vi "ttm_start.vi"() -> ()   [LabVIEW 2011]
panel:
  in  "ttm_twocreep_ramprate":dbl=0.001
  in  "ttm_twocreep_relaxationtime":dbl=30.0
  in  "ttm_twocreep_loadtime":dbl=30.0
  in  "ttm_twocreep_load":dbl=0.01
  in  "ttm_movetosetpoint_setpointtime":dbl=5.0
  in  "ttm_movetosetpoint_rampsetpoint":dbl
  in  "ttm_tensile_ramprate":dbl=0.01 step=0.001
  in  "ttm_tensile_rampamplitude":dbl=5000.0
  in  "ttm_tensile_channel":i32=1
  in  "ttm_aecontrol_channel":i32=1
  in  "ttm_aecontrol_rampratesilent":dbl=0.01 step=0.001
  in  "ttm_aecontrol_holdtime":dbl=5000.0
  in  "ttm_aecontrol_timewindow":dbl=1000.0
  in  "ttm_tensilecyclic_channel":dbl=1.0
  in  "ttm_tensilecyclic_separateloggings":bool=TRUE
  in  "ttm_tensilecyclic_ramptargetpressure":dbl=-700.0
  in  "ttm_tensilecyclic_zdim3":dbl=11.1
  in  "ttm_tensilecyclic_ydim3":dbl=11.1
  in  "ttm_tensilecyclic_xdim3":dbl=11.1
  in  "ttm_tensilecyclic_zdim2":dbl=11.1
  in  "ttm_tensilecyclic_ydim2":dbl=11.1
  in  "ttm_tensilecyclic_xdim2":dbl=11.1
  in  "ttm_tensilecyclic_zdim1":dbl=11.1
  in  "ttm_tensilecyclic_ydim1":dbl=11.1
  in  "ttm_tensilecyclic_xdim1":dbl=11.1
  in  "ttm_global_comment":string
  in  "ttm_tensilecyclic_timecycles":i32=10
  in  "ttm_tensilecyclic_timepreramp":i32=5
  in  "ttm_tensilecyclic_rampsetpoint":dbl=-0.04
  in  "ttm_tensilecyclic_numberofrounds":i32=2
  in  "ttm_tensilecyclic_cyclicfrequency":dbl=0.5
  in  "ttm_tensilecyclic_cyclicamplitude":dbl=0.05
  in  "ttm_global_expid":string="test"
  in  "ttm_global_parentfolder":string="C:\\Documents and Settings\\sauna\\Desktop\\MatleenaLabVIEW\\Testing\\"
  in  "ttm_aecontrol_targetvalue":dbl=1.0
  in  "aechangeofforcewithinbufferloop":dbl
  in  "ttm_aecontrol_aedatasum":dbl
  in  "ttm_aecontrol_initialforce":dbl
  in  "ttm_global_window":dbl
  in  "ttm_creep_channel":dbl=1.0
  in  "ttm_tensilecyclic_cyclicsetpoint":dbl=-0.1
  in  "ttm_aecontrol_ramprateae":dbl
  in  "ttm_global_protocol":string="tensilecyclic"
  in  "ttm_creep_load":dbl
  in  "ttm_tensilecyclic_ramprate":dbl=-0.01
  # "* = \"Put this negative if you are doing a compression experiment.\""
  # "*\n*\n*\n*\n*\n*\n*\n*\n*\n*\n*\n*\n*\n*\n*\n*\n*\n*\n*\n*"
  # "*"
  # "*"
  # "*"
  # "*"
  # "MEASUREMENTS AS MILLIMETERS"
  # "NOTE! \nDO NOT use double dots! (:)"
  # "***************************************"
  # "*\n*\n*\n*\n*\n*\n*\n*\n*\n*\n*\n*\n*\n*\n*"
  # "<-- \nPut negative values in these two  if you want to make compression (upper plate moving down).\n<---"
  # "<-- Separate ramp parts and cyclic parts into separate files"
  # "<-- Put all the data into the same file"
  # "***************************************"
  # "***************************************"
  # "*******************************"
  # "*\n*\n*\n*\n*\n*\n*\n*\n*\n*\n*\n*\n*\n*\n*"
  # "AE CONTROL"
  # "***************************************"
  # "mm/s"
  # "mm/s"
  # "ms"
  # "ms"
  # "AE control DEPRECATED?"
  # "How many events are needed within timewindow before changing to ramprateae"
  # "This actually is calculated in AE_data_read, initial value should be 0"
  # "1=position, 2=load, 3=digital position"
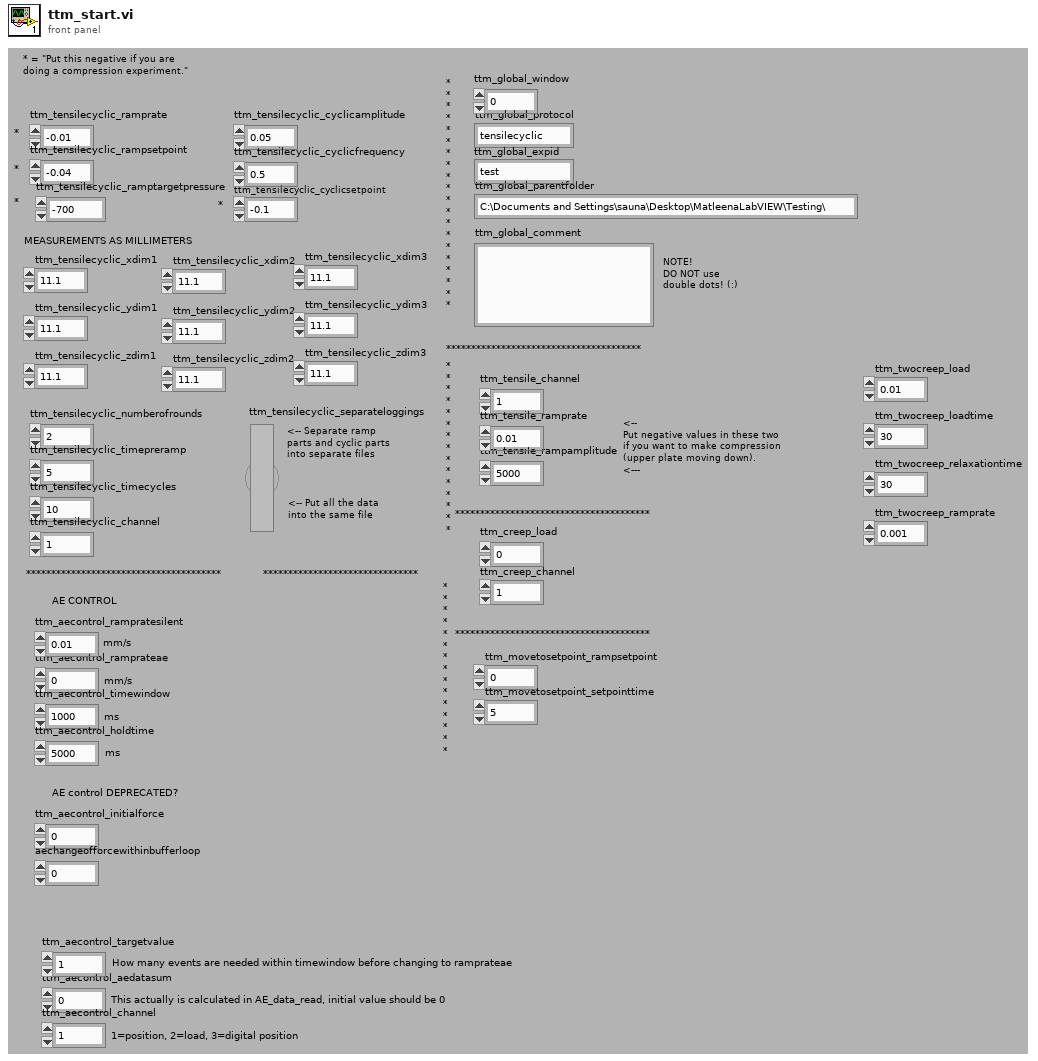
[diagram p1: front panel]
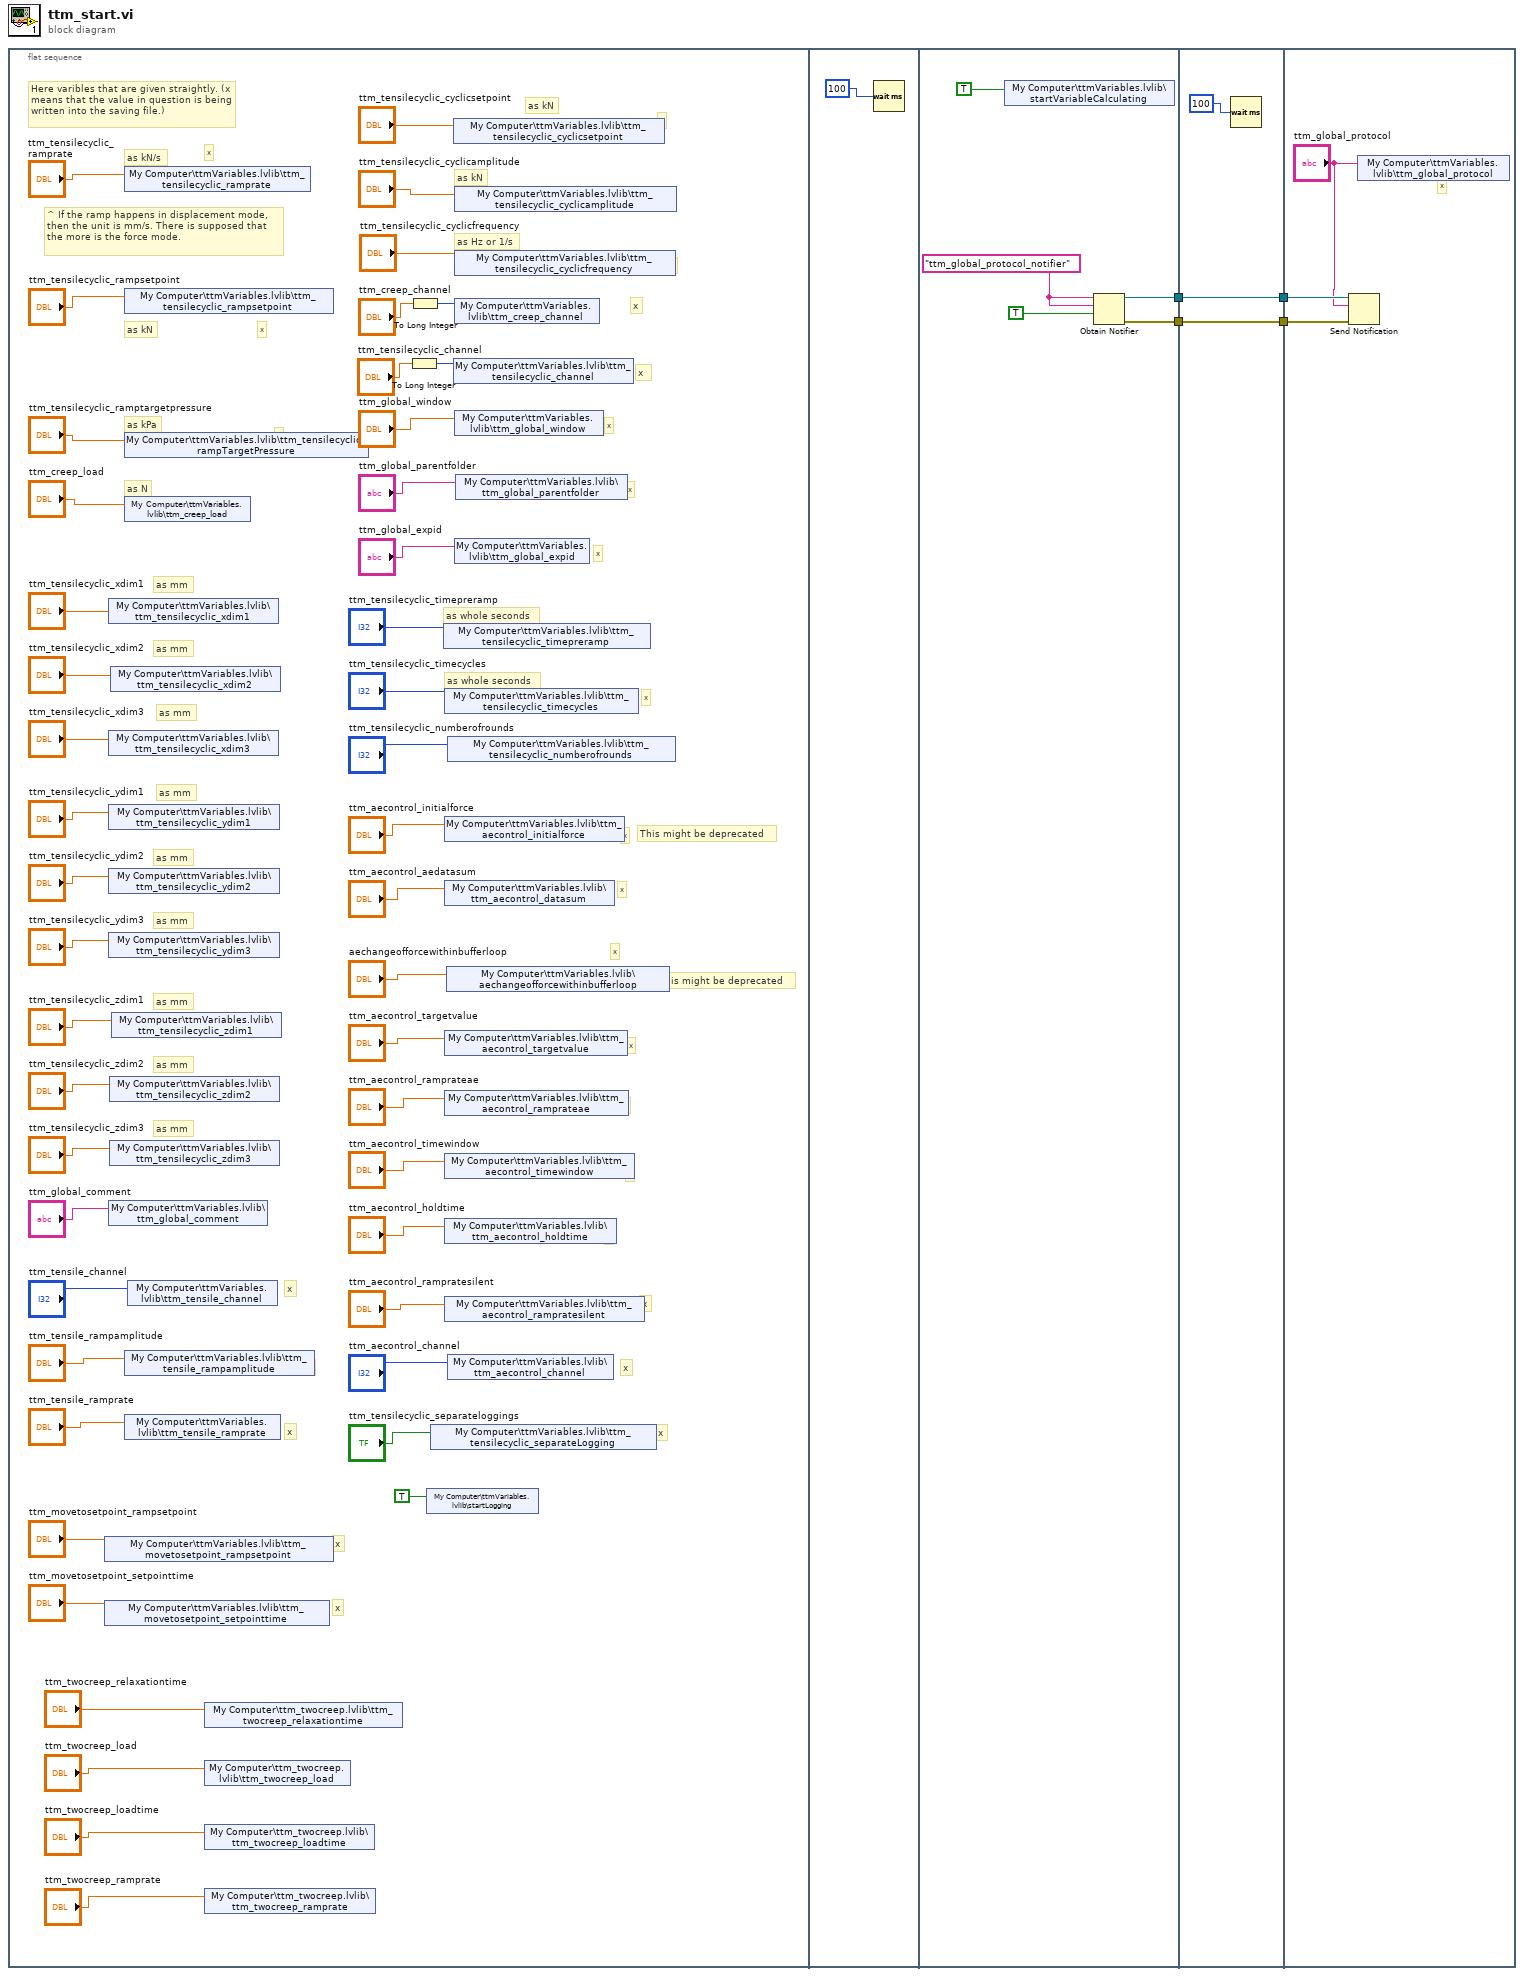
[diagram p0: block diagram]
diagram:
  n1 = flat-sequence {
    tunnel: [w54] -> w3
    tunnel: [w53] -> w1
    tunnel: [w59] -> w4
    tunnel: w3 -> [w59]
    tunnel: [w58] -> w2
    tunnel: w1 -> [w58]
    tunnel: w4 -> [w63]
    tunnel: w2 -> [w61]
    frame #0 {
      # "x"
      # "x"
      # "x"
      # "x"
      # "x"
      # "x"
      # "x"
      # "This might be deprecated"
      # "x"
      # "x"
      # "x"
      # "This might be deprecated"
      # "x"
      # "^ If the ramp happens in displacement mode, then the unit is mm/s. There is supposed that the more is the force mode."
      # "as kN"
      # "as Hz or 1/s"
      # "as N"
      # "as kN"
      # "as kN/s"
      # "as mm"
      # "as mm"
      # "as mm"
      # "as mm"
      # "as mm"
      # "as mm"
      # "as mm"
      # "as mm"
      # "as mm"
      # "as kN"
      # "as whole seconds"
      # "as whole seconds"
      # "Here varibles that are given straightly. (x means that the value in question is being written into the saving file.)"
      # "x"
      # "as kPa"
      # "x"
      # "x"
      # "x"
      # "x"
      # "x"
      # "x"
      # "x"
      # "x"
      # "x"
      # "x"
      # "x"
      # "x"
      # "x"
      # "x"
      # "x"
      # "x"
      # "x"
      # "x"
      # "x"
      n2 = shared-variable "My Computer\\ttmVariables.lvlib\\ttm_movetosetpoint_rampsetpoint"("ttm_movetosetpoint_rampsetpoint") -> ()  [unwired: 1 in, 1 out]
      n3 = shared-variable "My Computer\\ttmVariables.lvlib\\ttm_movetosetpoint_setpointtime"("ttm_movetosetpoint_setpointtime") -> ()  [unwired: 1 in, 1 out]
      n4 = shared-variable "My Computer\\ttmVariables.lvlib\\ttm_tensilecyclic_xdim1"("ttm_tensilecyclic_xdim1") -> ()  [unwired: 1 in, 1 out]
      n5 = shared-variable "My Computer\\ttmVariables.lvlib\\ttm_tensilecyclic_xdim3"("ttm_tensilecyclic_xdim3") -> ()  [unwired: 1 in, 1 out]
      n6 = shared-variable "My Computer\\ttmVariables.lvlib\\ttm_tensilecyclic_ydim1"("ttm_tensilecyclic_ydim1") -> ()  [unwired: 1 in, 1 out]
      n7 = shared-variable "My Computer\\ttmVariables.lvlib\\ttm_tensilecyclic_ydim2"("ttm_tensilecyclic_ydim2") -> ()  [unwired: 1 in, 1 out]
      n8 = shared-variable "My Computer\\ttmVariables.lvlib\\ttm_tensilecyclic_ydim3"("ttm_tensilecyclic_ydim3") -> ()  [unwired: 1 in, 1 out]
      n9 = shared-variable "My Computer\\ttmVariables.lvlib\\ttm_global_comment"("ttm_global_comment") -> ()  [unwired: 1 in, 1 out]
      n10 = shared-variable "My Computer\\ttmVariables.lvlib\\ttm_tensilecyclic_zdim2"("ttm_tensilecyclic_zdim2") -> ()  [unwired: 1 in, 1 out]
      n11 = shared-variable "My Computer\\ttmVariables.lvlib\\ttm_tensilecyclic_zdim3"("ttm_tensilecyclic_zdim3") -> ()  [unwired: 1 in, 1 out]
      n12 = shared-variable "My Computer\\ttmVariables.lvlib\\ttm_tensilecyclic_xdim2"("ttm_tensilecyclic_xdim2") -> ()  [unwired: 1 in, 1 out]
      n13 = shared-variable "My Computer\\ttmVariables.lvlib\\ttm_tensilecyclic_zdim1"("ttm_tensilecyclic_zdim1") -> ()  [unwired: 1 in, 1 out]
      n14 = shared-variable "My Computer\\ttmVariables.lvlib\\ttm_tensilecyclic_ramprate"("ttm_tensilecyclic_ramprate") -> ()  [unwired: 1 in, 1 out]
      n15 = shared-variable "My Computer\\ttmVariables.lvlib\\ttm_tensilecyclic_rampsetpoint"("ttm_tensilecyclic_rampsetpoint") -> ()  [unwired: 1 in, 1 out]
      n16 = shared-variable "My Computer\\ttmVariables.lvlib\\ttm_tensilecyclic_rampTargetPressure"("ttm_tensilecyclic_ramptargetpressure") -> ()  [unwired: 1 in, 1 out]
      n17 = shared-variable "My Computer\\ttmVariables.lvlib\\ttm_creep_load"("ttm_creep_load") -> ()  [unwired: 1 in, 1 out]
      n18 = shared-variable "My Computer\\ttmVariables.lvlib\\ttm_tensile_rampamplitude"("ttm_tensile_rampamplitude") -> ()  [unwired: 1 in, 1 out]
      n19 = shared-variable "My Computer\\ttmVariables.lvlib\\ttm_tensile_ramprate"("ttm_tensile_ramprate") -> ()  [unwired: 1 in, 1 out]
      n20 = shared-variable "My Computer\\ttmVariables.lvlib\\ttm_tensile_channel"("ttm_tensile_channel") -> ()  [unwired: 1 in, 1 out]
      n21 = shared-variable "My Computer\\ttm_twocreep.lvlib\\ttm_twocreep_relaxationtime"("ttm_twocreep_relaxationtime") -> ()  [unwired: 1 in, 1 out]
      n22 = shared-variable "My Computer\\ttm_twocreep.lvlib\\ttm_twocreep_load"("ttm_twocreep_load") -> ()  [unwired: 1 in, 1 out]
      n23 = shared-variable "My Computer\\ttm_twocreep.lvlib\\ttm_twocreep_loadtime"("ttm_twocreep_loadtime") -> ()  [unwired: 1 in, 1 out]
      n24 = shared-variable "My Computer\\ttm_twocreep.lvlib\\ttm_twocreep_ramprate"("ttm_twocreep_ramprate") -> ()  [unwired: 1 in, 1 out]
      n25 = To Long Integer(number="ttm_tensilecyclic_channel") -> (32bit integer=w19:i32)
      n26 = To Long Integer(number="ttm_creep_channel") -> (32bit integer=w32:i32)
      n27 = shared-variable "My Computer\\ttmVariables.lvlib\\startLogging"(TRUE ("startLogging")) -> ()  [unwired: 1 in, 1 out]
      n28 = shared-variable "My Computer\\ttmVariables.lvlib\\ttm_tensilecyclic_separateLogging"("ttm_tensilecyclic_separateloggings") -> ()  [unwired: 1 in, 1 out]
      n29 = shared-variable "My Computer\\ttmVariables.lvlib\\ttm_tensilecyclic_timepreramp"("ttm_tensilecyclic_timepreramp") -> ()  [unwired: 1 in, 1 out]
      n30 = shared-variable "My Computer\\ttmVariables.lvlib\\ttm_tensilecyclic_timecycles"("ttm_tensilecyclic_timecycles") -> ()  [unwired: 1 in, 1 out]
      n31 = shared-variable "My Computer\\ttmVariables.lvlib\\ttm_aecontrol_initialforce"("ttm_aecontrol_initialforce") -> ()  [unwired: 1 in, 1 out]
      n32 = shared-variable "My Computer\\ttmVariables.lvlib\\ttm_aecontrol_datasum"("ttm_aecontrol_aedatasum") -> ()  [unwired: 1 in, 1 out]
      n33 = shared-variable "My Computer\\ttmVariables.lvlib\\ttm_aecontrol_targetvalue"("ttm_aecontrol_targetvalue") -> ()  [unwired: 1 in, 1 out]
      n34 = shared-variable "My Computer\\ttmVariables.lvlib\\ttm_aecontrol_ramprateae"("ttm_aecontrol_ramprateae") -> ()  [unwired: 1 in, 1 out]
      n35 = shared-variable "My Computer\\ttmVariables.lvlib\\ttm_aecontrol_timewindow"("ttm_aecontrol_timewindow") -> ()  [unwired: 1 in, 1 out]
      n36 = shared-variable "My Computer\\ttmVariables.lvlib\\ttm_aecontrol_holdtime"("ttm_aecontrol_holdtime") -> ()  [unwired: 1 in, 1 out]
      n37 = shared-variable "My Computer\\ttmVariables.lvlib\\ttm_aecontrol_rampratesilent"("ttm_aecontrol_rampratesilent") -> ()  [unwired: 1 in, 1 out]
      n38 = shared-variable "My Computer\\ttmVariables.lvlib\\aechangeofforcewithinbufferloop"("aechangeofforcewithinbufferloop") -> ()  [unwired: 1 in, 1 out]
      n39 = shared-variable "My Computer\\ttmVariables.lvlib\\ttm_tensilecyclic_numberofrounds"("ttm_tensilecyclic_numberofrounds") -> ()  [unwired: 1 in, 1 out]
      n40 = shared-variable "My Computer\\ttmVariables.lvlib\\ttm_aecontrol_channel"("ttm_aecontrol_channel") -> ()  [unwired: 1 in, 1 out]
      n41 = shared-variable "My Computer\\ttmVariables.lvlib\\ttm_tensilecyclic_cyclicsetpoint"("ttm_tensilecyclic_cyclicsetpoint") -> ()  [unwired: 1 in, 1 out]
      n42 = shared-variable "My Computer\\ttmVariables.lvlib\\ttm_tensilecyclic_channel"(w19) -> ()  [unwired: 1 in, 1 out]
      n43 = shared-variable "My Computer\\ttmVariables.lvlib\\ttm_tensilecyclic_cyclicamplitude"("ttm_tensilecyclic_cyclicamplitude") -> ()  [unwired: 1 in, 1 out]
      n44 = shared-variable "My Computer\\ttmVariables.lvlib\\ttm_tensilecyclic_cyclicfrequency"("ttm_tensilecyclic_cyclicfrequency") -> ()  [unwired: 1 in, 1 out]
      n45 = shared-variable "My Computer\\ttmVariables.lvlib\\ttm_creep_channel"(w32) -> ()  [unwired: 1 in, 1 out]
      n46 = shared-variable "My Computer\\ttmVariables.lvlib\\ttm_global_window"("ttm_global_window") -> ()  [unwired: 1 in, 1 out]
      n47 = shared-variable "My Computer\\ttmVariables.lvlib\\ttm_global_expid"("ttm_global_expid") -> ()  [unwired: 1 in, 1 out]
      n48 = shared-variable "My Computer\\ttmVariables.lvlib\\ttm_global_parentfolder"("ttm_global_parentfolder") -> ()  [unwired: 1 in, 1 out]
    }
    frame #1 {
      n49 = Wait (ms)(milliseconds to wait=u32 100) -> ()  [unwired: 1 out]
    }
    frame #2 {
      w56 = "ttm_global_protocol_notifier" ("name (unnamed)")
      n50 = shared-variable "My Computer\\ttmVariables.lvlib\\startVariableCalculating"(TRUE ("startLogging")) -> ()  [unwired: 1 in, 1 out]
      n51 = Obtain Notifier(name (unnamed)=w56, notification data type=w56, create if not found? (T)=TRUE) -> (notifier out=w54:refnum<notifier>, error out=w53:errorcluster)  [unwired: 1 in, 1 out]
    }
    frame #3 {
      n52 = Wait (ms)(milliseconds to wait=u32 100) -> ()  [unwired: 1 out]
    }
    frame #4 {
      # "x"
      n53 = Send Notification(notification="ttm_global_protocol", notifier=w63, error in (no error)=w61) -> ()  [unwired: 2 out]
      n54 = shared-variable "My Computer\\ttmVariables.lvlib\\ttm_global_protocol"("ttm_global_protocol") -> ()  [unwired: 1 in, 1 out]
    }
  }
